vi "Save_to_Project.vi"(8 "error in (no error)":errorcluster, 9 "index":i32, 10 "buildObject":T1, 11 "AB_Source_VI in":refnum<class "AB_Source_VI.lvclass">) -> (0 "error out":errorcluster, 3 "AB_Source_VI out":refnum<class "AB_Source_VI.lvclass">)   [LabVIEW 2020, in "AB_Source_VI.lvclass"]
uses:
  <vilib>/AppBuilder/AB_Classes/Source/VI/AB_Source_VI.lvclass
  <resource>/Framework/Providers/API/ItemRef.ctl
  <vilib>/AppBuilder/RW_Project/AB_RW_Project_Source_VI_Data.ctl
  <vilib>/AppBuilder/RW_Project/AB_RW_Project_PropBag_Action.ctl
  <vilib>/AppBuilder/AB_Classes/Source/VI/AB_Source_VI.lvclass/AB_Source_VI.ctl
  <vilib>/AppBuilder/AB_Classes/Source/AB_Source.lvclass
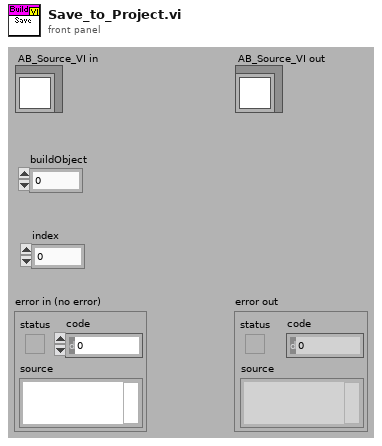
[diagram p1: front panel]
types:
  T1 = typedef "ItemRef.ctl" = u64
  T2 = typedef "AB_RW_Project_Source_VI_Data.ctl" = cluster{"LLBtopLevel":bool, "privateDataControl":bool}
  T3 = typedef "AB_RW_Project_PropBag_Action.ctl" = enum16{"read", "write", "clear", "readPrevious", "writePrevious", "clearPrevious"}
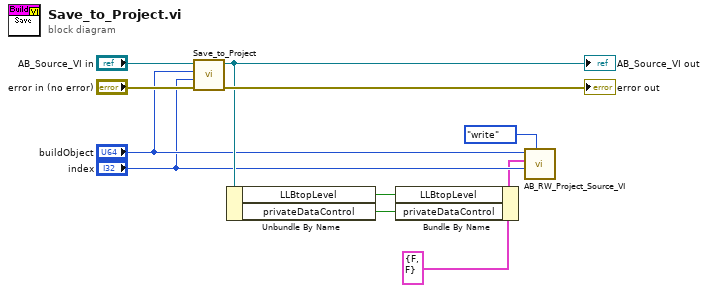
[diagram p0: block diagram]
diagram:
  n1 = call-parent "Save_to_Project.vi"("error in (no error)"="error in (no error)", "index"="index", "buildObject"="buildObject", "AB_Source in"="AB_Source_VI in") -> ("error out"=→"error out":errorcluster, "AB_Source out"=w8:refnum<class "AB_Source_VI.lvclass">)  [unwired: 6 in]
  "AB_Source_VI out" <- w8
  n2 = Unbundle By Name(w8) -> ("LLBtopLevel"=w2:bool, "privateDataControl"=w1:bool)
  n3 = Bundle By Name(cluster=T2 {"LLBtopLevel"=FALSE, "privateDataControl"=FALSE} ("dataSource in"), "LLBtopLevel"=w2, "privateDataControl"=w1) -> (w3:T2)
  n4 = call <vilib>:"AB_RW_Project_Source_VI.vi"("action"=AB_RW_Project_PropBag_Action."write", "index in"="index", "dataSource in"=w3, "buildObject"="buildObject") -> ()  [unwired: 4 in, 4 out]
